vi "Write Digital Transition Type.vi"(5 "Digital Transition Type":u8, 9 "Plot in":refnum<class "Plot.lvclass">) -> (3 "Plot out":refnum<class "Plot.lvclass">)   [LabVIEW 2014, in "Plot.lvclass"]
uses:
  Plot.lvclass
  Plot.lvclass/Plot.ctl
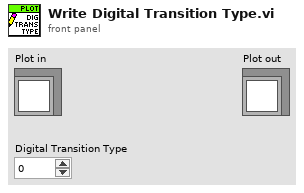
[diagram p1: front panel]
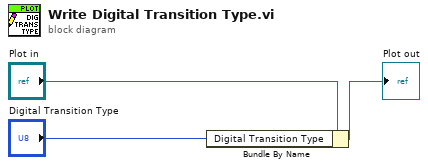
[diagram p0: block diagram]
diagram:
  n1 = Bundle By Name(cluster="Plot in", "Digital Transition Type"="Digital Transition Type") -> (→"Plot out":refnum<class "Plot.lvclass">)
